vi "Read T.vi"(11 "HE1_Z_state in":refnum<class "HE_Z_state.lvclass">) -> (2 "T (ms)":u32, 3 "HE1_Z_state out":refnum<class "HE_Z_state.lvclass">)   [LabVIEW 2019, in "Heating.lvlib" / "HE_Z_state.lvclass"]
uses:
  HE_Z_state.lvclass
  D:/my_projects/projects/Algorithms/Labview/19/Sequence/State/State.lvclass
  Sequence/State/State.lvclass/State.ctl
  Sequence/State/State.lvclass
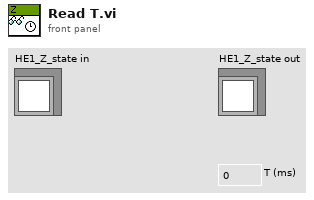
[diagram p1: front panel]
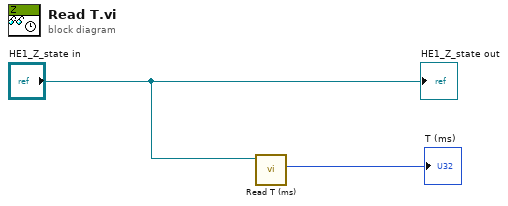
[diagram p0: block diagram]
diagram:
  n1 = call "Read T (ms).vi"("State in"="HE1_Z_state in") -> ("T (ms)"=→"T (ms)":u32)  [unwired: 9 in, 1 out]
  "HE1_Z_state out" <- "HE1_Z_state in"
